vi "CheezyMsatan.vi"(1 "arg":dbl) -> (0 "msatan(arg)":dbl)   [LabVIEW 2016]
uses:
  <userlib>/836-Libraries/Math/CheezyMath/MathConstantsNames.ctl
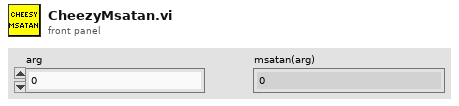
[diagram p1: front panel]
types:
  T1 = typedef "MathConstantsNames.ctl" = enum16{"sq2p1", "sq2m1", "p4", "p3", "p2", "p1", "p0", "q4", "q3", "q2", "q1", "q0", "PIO2"}
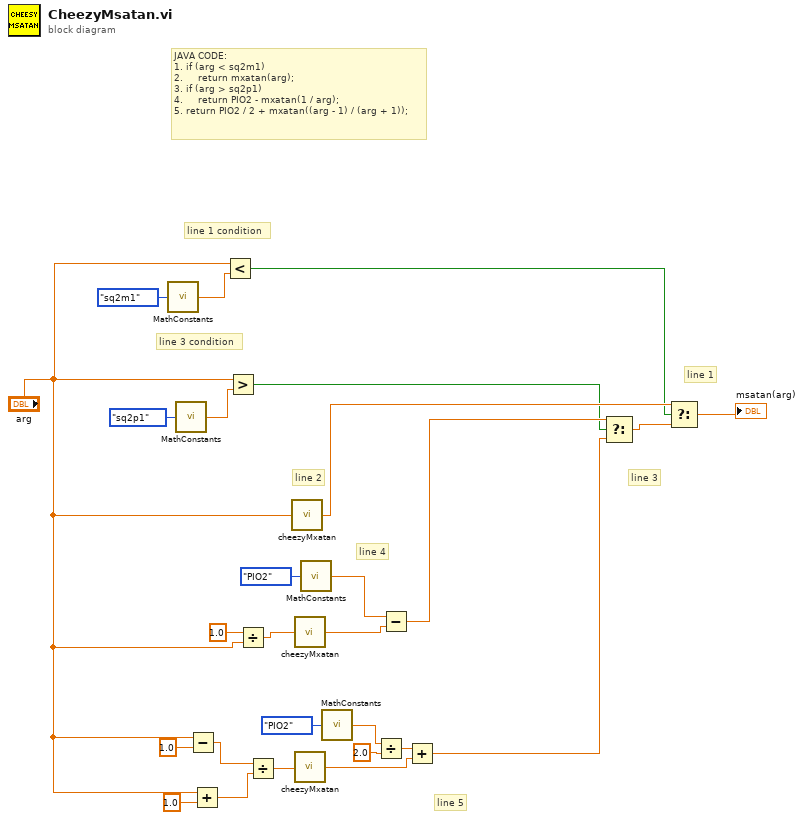
[diagram p0: block diagram]
diagram:
  # "line 5"
  # "line 3"
  # "line 1"
  # "line 4"
  # "line 2"
  # "line 3 condition"
  # "line 1 condition"
  # "JAVA CODE:\n1. if (arg < sq2m1)\n2.     return mxatan(arg);\n3. if (arg > sq2p1)\n4.     return PIO2 - mxatan(1 / arg);\n5. return PIO2 / 2 + mxatan((arg - 1) / (arg + 1));"
  n1 = call <userlib>:"MathConstants.vi"("Constant Name"=MathConstantsNames."sq2m1") -> ("Constant Value"=w26:dbl)
  n2 = call <userlib>:"MathConstants.vi"("Constant Name"=MathConstantsNames."sq2p1") -> ("Constant Value"=w25:dbl)
  n3 = Subtract(x="arg", y=1.0) -> (x-y=w15:dbl)
  n4 = Add(x="arg", y=1.0) -> (x+y=w14:dbl)
  n5 = Less?(x="arg", y=w26) -> (x < y?=w5:bool)
  n6 = Greater?(x="arg", y=w25) -> (0:w4:bool)
  n7 = Divide(x=1.0, y="arg") -> (x/y=w23:dbl)
  n8 = Divide(x=w15, y=w14) -> (x/y=w13:dbl)
  n9 = call <userlib>:"cheezyMxatan.vi"("arg"="arg") -> ("mxatan(arg)"=w6:dbl)
  n10 = call <userlib>:"cheezyMxatan.vi"("arg"=w23) -> ("mxatan(arg)"=w21:dbl)
  n11 = call <userlib>:"cheezyMxatan.vi"("arg"=w13) -> ("mxatan(arg)"=w1:dbl)
  n12 = call <userlib>:"MathConstants.vi"("Constant Name"=MathConstantsNames."PIO2") -> ("Constant Value"=w20:dbl)
  n13 = call <userlib>:"MathConstants.vi"("Constant Name"=MathConstantsNames."PIO2") -> ("Constant Value"=w12:dbl)
  n14 = Divide(x=w12, y=2.0) -> (x/y=w8:dbl)
  n15 = Subtract(x=w20, y=w21) -> (x-y=w7:dbl)
  n16 = Add(x=w8, y=w1) -> (x+y=w2:dbl)
  n17 = Select(t=w7, s=w4, f=w2) -> (s? t:f=w9:dbl)
  n18 = Select(t=w6, s=w5, f=w9) -> (s? t:f=→"msatan(arg)":dbl)
